vi "solar Msg Other (TLM-Broadcast).vi"(8 "error in (no error)":errorcluster, 9 "TLM_DATA":variant, 10 "TLM":string, 11 "solar in":refnum<class "solar.lvclass">) -> (0 "error out":errorcluster, 3 "solar out":refnum<class "solar.lvclass">)   [LabVIEW 2018]
doc: "This returns the Voyager telemetry and broadcasts the message to the subscribed queues and user events."
uses:
  solar.lvclass
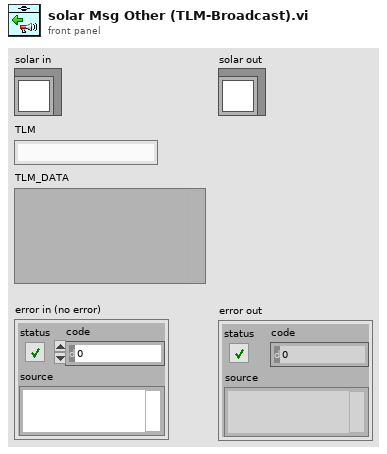
[diagram p1: front panel]
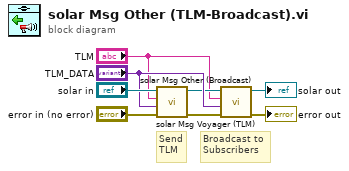
[diagram p0: block diagram]
diagram:
  # "Broadcast to\nSubscribers"
  # "Send\nTLM"
  n1 = call "solar Msg Voyager (TLM).vi"("error in (no error)"="error in (no error)", "TLM_DATA (No HDR)"="TLM_DATA", "TLM"="TLM", "solar in"="solar in") -> ("error out"=w3:errorcluster, "solar out"=w2:refnum<class "solar.lvclass">)  [unwired: 6 in]
  n2 = call "solar Msg Other (Broadcast).vi"("error in (no error)"=w3, "TLM_DATA"="TLM_DATA", "TLM"="TLM", "solar in"=w2) -> ("error out"=→"error out":errorcluster, "solar out"=→"solar out":refnum<class "solar.lvclass">)  [unwired: 6 in]
